vi "Set_Pxl_Format.vi"(8 "error in (no error)":errorcluster, 11 ".NET Refnum in":refnum<k24>) -> (0 "error out":errorcluster)   [LabVIEW 2021]
uses:
  C:/Program Files/Thorlabs/Scientific Imaging/ThorCam/uc480DotNet.dll
  Program Files/Thorlabs/Scientific Imaging/ThorCam/uc480DotNet.dll
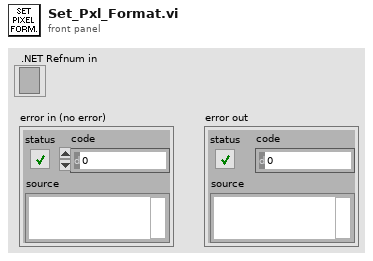
[diagram p1: front panel]
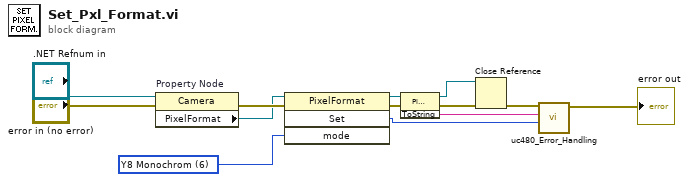
[diagram p0: block diagram]
diagram:
  w1 = 6 items=["RGB 32"=0, "RGB 24"=1, "Y8 Monochrom"=6] ("Mode")
  n1 = property on="Property Node" class="Camera"(reference=".NET Refnum in", error in="error in (no error)") -> (error out=w3:errorcluster, "PixelFormat"=w2:refnum<k24>)  [unwired: 1 out]
  n2 = invoke class="PixelFormat" method="Set"(reference=w2, error in=w3, "mode"=w1) -> (reference out=w6:refnum<k24>, error out=w8:errorcluster, "Set"=w7:i32)  [unwired: 1 in, 1 out]
  n3 = invoke class="PixelFormat" method="ToString"(reference=w6, error in=w8) -> (reference out=w10:refnum<k24>, error out=w9:errorcluster, "ToString"=w5:string)  [unwired: 1 in]
  n4 = Close Reference(reference=w10, error in (no error)=w9) -> (error out=w12:errorcluster)
  n5 = call "uc480_Error_Handling.vi"("Error Code"=w7, "Error String"=w5, "Error In"=w12) -> ("Error Out"=→"error out":errorcluster)  [unwired: 8 in]
